vi "LVOOP Return Class Name__ogtk.vi"(0 "Object":refnum<class>) -> (1 "Class Base Name":string, 2 "Qualified Name":string, 3 "Qualified Name Array":string[](array[string]))   [LabVIEW 2016]
doc: "Returns the <b>Class Base Name</b>, <b>Qualified Name</b> and <b>Qualified Name Array</b> of <b>Object</b>.\n\nFor example if <b>Object</b> is of type <b>Library.lvlib:Class 1.lvclass</b> then:\n<b>Class Base Name</b> = Class 1\n<b>Qualified Name</b> = Library.lvlib:Class 1.lvclass\n<b>Qualified Name Array</b> = [Library.lvlib, Class 1.lvclass]\n\n<b>Notes:</b>\nThis VI benefits from being generic (e.g. good for probes/scripting) however, is most likely inefficient to the cost of flattening the entire object data to a string (as is any VI that does this). Although this VI is optimised to only use the default object data.\n\n<b>The following alternative method is recommended for high performance applications:</b>\nAdd a dynamic dispatch method to the root Class (e.g. called \"Get Class Name.vi\") and override that VI at every level of the hierarchy to return a string constant of the desired name. This avoids the memory allocation and performance hit of the flattening to the string. An example of a use case is creating a by-name-lookup object hierarchy."
panel:
  # "Please visit http://www.OpenG.org to learn about the\nOpen Source LabVIEW software movement.\n\nNOTICE -- YOU MUST LEAVE THIS NOTICE IN PLACE.  PER THE TERMS OF THE LICENSE BELOW, YOU MAY SUBLICENSE THIS SOFTWARE \nIN ANY WAY THAT DOES NOT CONFLICT WITH THIS LICENSE.\n\n### BSD License (http://www.opensource.org/licenses/bsd-license.php) Begin ###\n \nCopyright (c) 2012, James David Powell <drjdpowell@gmail.com>\nCopyright (c) 2012, Jonathon Green <jg@jgcode.net>\n\nAll rights reserved.\n\nRedistribution and use in source and binary forms, with or without modification, are permitted provided that the following conditions are met:\n\n    * Redistributions of source code must retain the above copyright notice, this list of conditions and the following disclaimer.\n    * Redistributions in binary form must reproduce the above copyright notice, this list of conditions and the following disclaimer in the \n       documentation and/or other materials provided with the distribution.\n    * Neither the name of OpenG.org nor the names of its contributors may be used to endorse or promote products derived \n       from this software without specific prior written permission.\n\nTHIS SOFTWARE IS PROVIDED BY THE COPYRIGHT HOLDERS AND CONTRIBUTORS \"AS IS\" AND ANY EXPRESS OR IMPLIED WARRANTIES, \nINCLUDING, BUT NOT LIMITED TO, THE IMPLIED WARRANTIES OF MERCHANTABILITY AND FITNESS FOR A PARTICULAR PURPOSE ARE \nDISCLAIMED. IN NO EVENT SHALL THE COPYRIGHT OWNER OR CONTRIBUTORS BE LIABLE FOR ANY DIRECT, INDIRECT, INCIDENTAL,\n SPECIAL, EXEMPLARY, OR CONSEQUENTIAL DAMAGES (INCLUDING, BUT NOT LIMITED TO, PROCUREMENT OF SUBSTITUTE GOODS OR \nSERVICES; LOSS OF USE, DATA, OR PROFITS; OR BUSINESS INTERRUPTION) HOWEVER CAUSED AND ON ANY THEORY OF LIABILITY, \nWHETHER IN CONTRACT, STRICT LIABILITY, OR TORT (INCLUDING NEGLIGENCE OR OTHERWISE) ARISING IN ANY WAY OUT OF THE USE \nOF THIS SOFTWARE, EVEN IF ADVISED OF THE POSSIBILITY OF SUCH DAMAGE.\n\n### BSD License End ###"
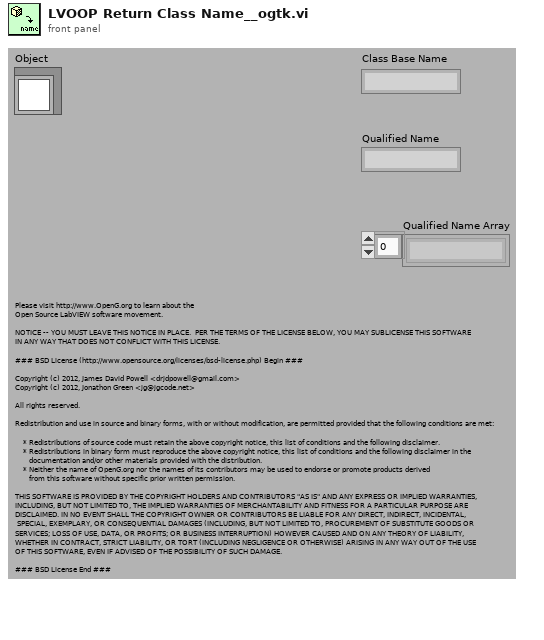
[diagram p1: front panel]
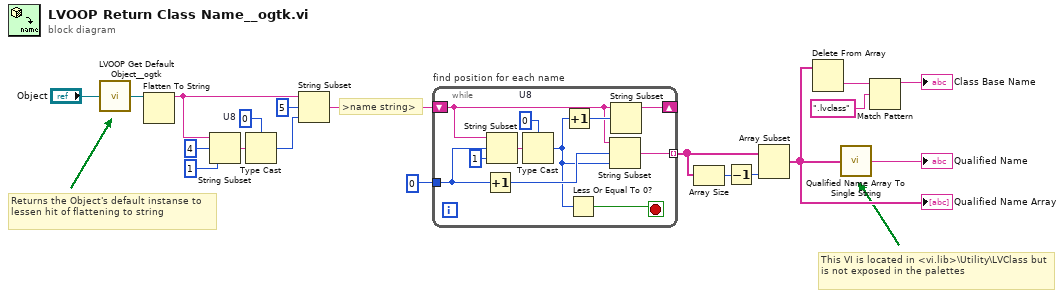
[diagram p0: block diagram]
diagram:
  w11 = u8 0  # U8
  # ">name string>"
  # "This VI is located in <vi.lib>\\Utility\\LVClass but is not exposed in the palettes"
  # "Returns the Object's default instanse to lessen hit of flattening to string"
  n1 = call "LVOOP Get Default Object__ogtk.vi"("Object"="Object") -> ("Object Default Instance"=w1:refnum<class>)
  n2 = Flatten To String(anything=w1) -> (data string=w3:string)  [unwired: 1 in, 4 out]
  n3 = String Subset(string=w3, offset (0)=4, length (rest)=1 ("length (rest)")) -> (substring=w12:string)
  n4 = Type Cast(type=w11, x=w12) -> (*(type *) &x=w9:u8)
  n5 = String Subset ("Name string")(string=w3, offset (0)=u8 5 ("y"), length (rest)=w9) -> (substring=w8:string)
  n6 = while "find position for each name" {
    shift-right: [w21] -> _
    shift-left: w8 -> [w22]
    tunnel: [w26] -> w7 mode=indexing
    tunnel: 0 ("offset (0)") -> [w20]
    stop <- w27 stop-if-true
    w30 = u8 0  # U8
    n7 = Increment(x=w20) -> (x+1=w25:i32)
    n8 = String Subset(string=w22, offset (0)=w20, length (rest)=1 ("length (rest)")) -> (substring=w29:string)
    n9 = Type Cast(type=w30, x=w29) -> (*(type *) &x=w24:u8)
    n10 = Increment(x=w24) -> (x+1=w23:u8)
    n11 = Less Or Equal To 0?(x=w24) -> (x <= 0?=w27:bool)
    n12 = String Subset(string=w22, offset (0)=w25, length (rest)=w24) -> (substring=w26:string)
    n13 = String Subset(string=w22, offset (0)=w23) -> (substring=w21:string)  [unwired: 1 in]
  }
  n14 = Array Size(array=w7) -> (size(s)=w6:i32)
  n15 = Decrement(x=w6) -> (x-1=w4:i32)
  n16 = Array Subset(array=w7, length=w4) -> (w2:string[])  [unwired: 1 in]
  "Qualified Name Array" <- w2
  n17 = Delete From Array(array=w2) -> (deleted portion=w18:string)  [unwired: 2 in, 1 out]
  n18 = call <vilib>:"Qualified Name Array To Single String.vi"("Fully Qualified Array"=w2) -> ("Fully Qualified String"=→"Qualified Name":string)
  n19 = Match Pattern(string=w18, regular expression=".lvclass") -> (before substring=→"Class Base Name":string)  [unwired: 1 in, 3 out]
